vi "final lunch menu sub vi.vi"() -> ()   [LabVIEW 2019]
uses:
  Program Files (x86)/National Instruments/LabVIEW 2019/project/EN1Course-master (12)/EN1Course-master/_Subs/ThingWorx/_TW_Subs/TW_XControl.xctl
  Program Files (x86)/National Instruments/LabVIEW 2019/project/EN1Course-master (12)/EN1Course-master/_Subs/ThingWorx/_TW_Subs/Thingworx_Write_string.vi
panel:
  in  "MadLGS":string(xcontrol)="Day1:MadLGS"
  in  "MadLP":string(xcontrol)="Day1:MadLP"
  in  "Mad1LV":string(xcontrol)="Day1:MadLV"
  in  "MadLE2":string(xcontrol)="Day1:MadLE2"
  in  "MadLE1":string(xcontrol)="Day1:MadLE1"
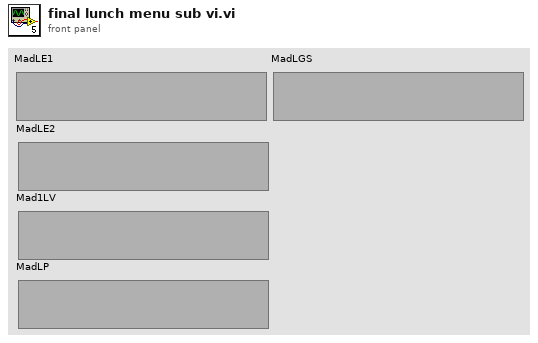
[diagram p1: front panel]
types:
  T1 = cluster{"menu-id":string, "data":cluster{"Lunch":cluster{"GRILLED SANDWICH":string[], "POTATO & RICE ACCOMPANIMENTS":string[], "VEGETABLES":string[], "LUNCH ENTREE":string[]}}}
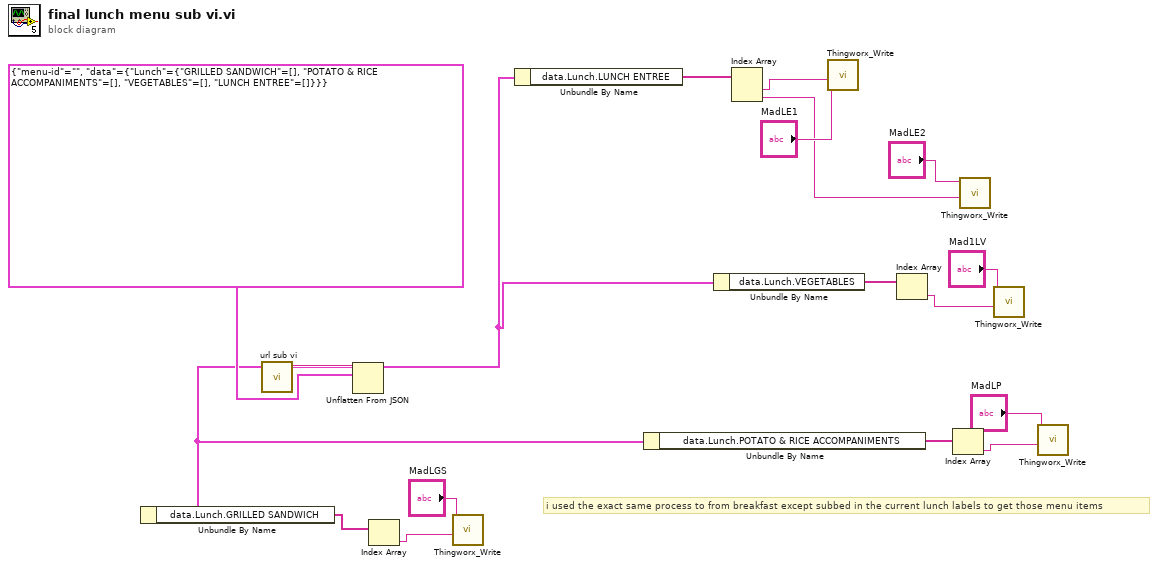
[diagram p0: block diagram]
diagram:
  # "i used the exact same process to from breakfast except subbed in the current lunch labels to get those menu items"
  n1 = call "url sub vi.vi"() -> ("body 2"=w17:string)  [unwired: 11 in]
  n2 = Unflatten From JSON(JSON string=w17, type and defaults=T1 {"menu-id"="", "data"={"Lunch"={"GRILLED SANDWICH"=[], "POTATO & RICE ACCOMPANIMENTS"=[], "VEGETABLES"=[], "LUNCH ENTREE"=[]}}}) -> (value=w15:T1)  [unwired: 5 in, 1 out]
  n3 = Unbundle By Name(w15) -> ("data.Lunch.GRILLED SANDWICH"=w14:string[])
  n4 = Index Array(array=w14) -> (element=w2:string)  [unwired: 1 in]
  n5 = call-poly "Thingworx_Write.vi"("String"=w2, "Thingworx"="MadLGS") -> ()  [unwired: 10 in]
  n6 = Unbundle By Name(w15) -> ("data.Lunch.LUNCH ENTREE"=w11:string[])
  n7 = Unbundle By Name(w15) -> ("data.Lunch.POTATO & RICE ACCOMPANIMENTS"=w13:string[])
  n8 = Unbundle By Name(w15) -> ("data.Lunch.VEGETABLES"=w12:string[])
  n9 = Index Array(array=w11) -> (element #1=w10:string, element #2=w8:string)  [unwired: 2 in]
  n10 = call-poly "Thingworx_Write.vi"("String"=w10, "Thingworx"="MadLE1") -> ()  [unwired: 10 in]
  n11 = Index Array(array=w12) -> (element=w6:string)  [unwired: 1 in]
  n12 = Index Array(array=w13) -> (element=w4:string)  [unwired: 1 in]
  n13 = call-poly "Thingworx_Write.vi"("String"=w8, "Thingworx"="MadLE2") -> ()  [unwired: 10 in]
  n14 = call-poly "Thingworx_Write.vi"("String"=w6, "Thingworx"="Mad1LV") -> ()  [unwired: 10 in]
  n15 = call-poly "Thingworx_Write.vi"("String"=w4, "Thingworx"="MadLP") -> ()  [unwired: 10 in]
